vi "oa_AC DC Separation Linear (1 Channel).vi"(7 "reset? (F)":bool, 8 "points/rev":u32, 9 "averaging revolution (1)":dbl=1.0 min=0.0, 10 "position info":T1, 11 "even angle signal":cluster{"r0":dbl, "dr":dbl, "Y":dbl[]}={"r0"=0.0, "dr"=1.0, "Y"=[]} {"r0" format="%.2p"; "dr" format="%.2p"; "Y" format="%.2f"}) -> (0 "DC even angle signal":cluster{"r0":dbl, "dr":dbl, "Y":dbl[]}, 1 "AC even angle signal":cluster{"r0":dbl, "dr":dbl, "Y":dbl[]}, 2 "position info out":T1, 3 "dul even angle signal":cluster{"r0":dbl, "dr":dbl, "Y":dbl[]})   [LabVIEW 2017, in "SoundVib_OAUtility.lvlib"]
uses:
  <vilib>/addons/Sound and Vibration/Order Analysis/Utility/SoundVib_OAUtility.lvlib
  <vilib>/addons/Sound and Vibration/Order Analysis/Misc/OAT Position Info.ctl
  <vilib>/Analysis/baseanly.llb/Mean (DBL).vi
  <vilib>/Analysis/NI_AALBase.lvlib
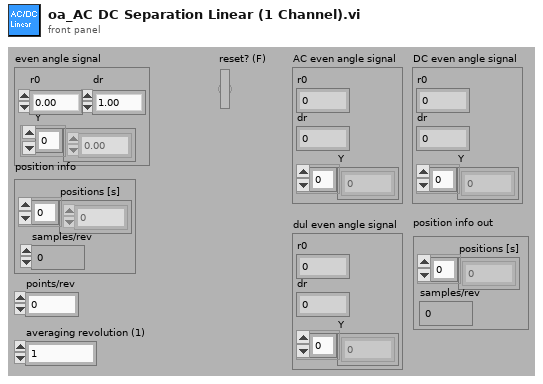
[diagram p1: front panel]
types:
  T1 = typedef "OAT Position Info.ctl" = cluster{"positions [s]":dbl[], "samples/rev":dbl}
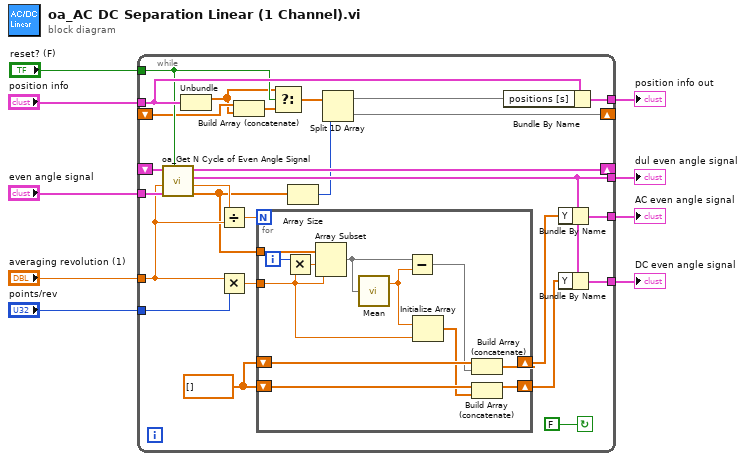
[diagram p0: block diagram]
diagram:
  n1 = while {
    tunnel: "reset? (F)" -> [w15]
    tunnel: "even angle signal" -> [w29]
    shift-right: [w28] -> _
    shift-left: _ -> [w30]
    tunnel: [w33] -> w6
    tunnel: [w31] -> w5
    tunnel: "points/rev" -> [w23]
    tunnel: [w26] -> w4
    tunnel: "averaging revolution (1)" -> [w21]
    tunnel: "position info" -> [w18]
    tunnel: [w16] -> w1
    shift-right: [w14] -> _
    shift-left: _ -> [w13]
    stop <- FALSE continue-if-true
    w27 = dbl[] [] ("second subarray")
    n2 = call <vilib>:"oa_Get N Cycle of Even Angle Signal.vi"("reset"=w15, "new even angle signal"=w29, "averaging revolution (1)"=w21, "rest even angle signal"=w30) -> ("data for averaging"=w19:dbl[], "number of averages"=w24:dbl, "even angle signal"=w26:cluster{"r0":dbl, "dr":dbl, "Y":dbl[]}, "rest even angle signal out"=w28:cluster{"r0":dbl, "dr":dbl, "Y":dbl[]})  [unwired: 4 in]
    n3 = Unbundle(w18) -> ("positions [s]"=w11:dbl[])  [unwired: 1 out]
    n4 = Divide(x=w24, y=w21) -> (x/y=w22:dbl)
    n5 = Multiply(x=w21, y=w23) -> (x*y=w25:dbl)
    n6 = Build Array (concatenate)(w13, w11) -> (w12:dbl[])
    n7 = for {
      N: w22 -> [_]
      tunnel: w25 -> [w38]
      shift-right: [w45] -> w34
      shift-left: w27 -> [w47]
      shift-right: [w41] -> w32
      shift-left: w27 -> [w43]
      tunnel: w19 -> [w40]
      i -> [w39]
      n8 = Multiply(x=w39, y=w38) -> (x*y=w37:dbl)
      n9 = Array Subset(array=w40, index=w37, length=w38) -> (w36:dbl[])
      n10 = call-poly <vilib>:"Mean.vi"("X"=w36) -> ("mean"=w44:dbl)  [unwired: 1 out]
      n11 = Subtract(x=w36, y=w44) -> (x-y=w46:dbl[])
      n12 = Initialize Array(w44, w38) -> (w42:dbl[])
      n13 = Build Array (concatenate)(w47, w46) -> (w45:dbl[])
      n14 = Build Array (concatenate)(w43, w42) -> (w41:dbl[])
    }
    n15 = Select(t=w11, s=w15, f=w12) -> (s? t:f=w10:dbl[])
    n16 = Array Size(array=w19) -> (size(s)=w20:i32)
    n17 = Split 1D Array(array=w10, index=w20) -> (first subarray=w17:dbl[], second subarray=w14:dbl[])
    n18 = Bundle By Name(cluster=w18, "positions [s]"=w17) -> (w16:T1)
    n19 = Bundle By Name(cluster=w26, "Y"=w34) -> (w33:cluster{"r0":dbl, "dr":dbl, "Y":dbl[]})
    n20 = Bundle By Name(cluster=w26, "Y"=w32) -> (w31:cluster{"r0":dbl, "dr":dbl, "Y":dbl[]})
  }
  "AC even angle signal" <- w6
  "DC even angle signal" <- w5
  "dul even angle signal" <- w4
  "position info out" <- w1
